vi "ControlReadPulseAll.vi"() -> (0 "PosOut":dbl[](array[numeric]))   [LabVIEW 2018]
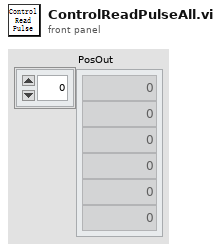
[diagram p1: front panel]
types:
  T1 = typedef "衰减片电机位置枚举器.ctl" = enum16{"0倍", "10倍", "100倍", "1000倍"}
  T2 = cluster{"激光器型号":string, "X":dbl, "Y":dbl, "Z":dbl, "Rotate":dbl, "Pitching":dbl, "DivergeAngle":dbl, "衰减片位置":cluster{"小积分球位置":T1, "偏振仪位置 ":T1, "近场相机位置 ":T1, "远场相机位置":T1}, "Type":string, "Serial":string}
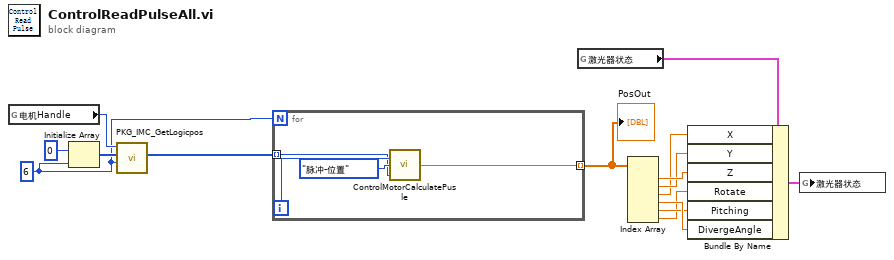
[diagram p0: block diagram]
diagram:
  w9 = 6 ("维数大小")
  n1 = global read "参数.vi" "电机Handle"() -> (w10:u32)
  n2 = Initialize Array(u32 0 ("元素"), w9) -> (w11:u32[])
  n3 = call "PKG_IMC_GetLogicpos.vi"("axisnum"=w9, "pos"=w11, "Handle"=w10) -> ("pos out"=w8:i32[])  [unwired: 6 in, 2 out]
  n4 = for {
    N: w9 -> [_]
    tunnel: [w17] -> w7 mode=indexing
    tunnel: w8 -> [w15] mode=indexing
    i -> [w16]
    n5 = call "ControlMotorCalculatePusle.vi"("数据"=w15, "计算状态"=enum32{"位置-脉冲", "脉冲-位置"}."脉冲-位置", "控制电机"=w16) -> ("dataout"=w17:dbl)  [unwired: 2 in]
  }
  "PosOut" <- w7
  n6 = global read "参数.vi" "激光器状态"() -> (w13:T2)
  n7 = Index Array(array=w7) -> (element #1=w6:dbl, element #2=w5:dbl, element #3=w4:dbl, element #4=w3:dbl, element #5=w2:dbl, element #6=w1:dbl)  [unwired: 6 in]
  n8 = Bundle By Name(cluster=w13, "X"=w4, "Y"=w5, "Z"=w6, "Rotate"=w1, "Pitching"=w2, "DivergeAngle"=w3) -> (w12:T2)
  n9 = global write "参数.vi" "激光器状态"(w12) -> ()
